vi "getClaseEstadistica.vi"(0 "claseEstadistica in":refnum<class "claseEstadistica.lvclass">, 3 "error in":errorcluster) -> (7 "claseEstadistica out":refnum<class "claseEstadistica.lvclass">, 8 "dataReading":T1, 10 "error out":errorcluster)   [LabVIEW 2014, in "claseEstadistica.lvclass"]
uses:
  claseEstadistica.lvclass
  claseEstadistica.lvclass/claseEstadistica.ctl
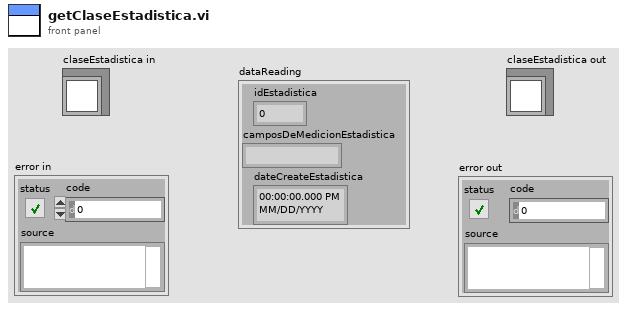
[diagram p1: front panel]
types:
  T1 = cluster{"idEstadistica":dbl, "camposDeMedicionEstadistica":string, "dateCreateEstadistica":timestamp}
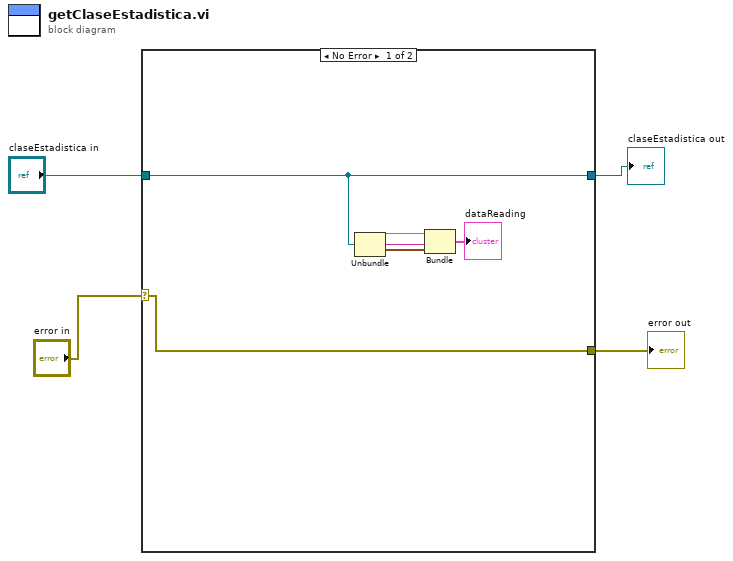
[diagram p0: block diagram]
diagram:
  n1 = case shown="No Error" "error in" {
    selector: "error in" -> [w10 w12]
    tunnel: [w10 w12] -> w3
    tunnel: "claseEstadistica in" -> [w9 w11]
    tunnel: [w9 w11] -> w1
    frame No Error {
      n2 = Unbundle(w9) -> (w8:dbl, w7:string, w6:timestamp)
      n3 = Bundle("idEstadistica"=w8, "camposDeMedicionEstadistica"=w7, "dateCreateEstadistica"=w6) -> (→"dataReading":T1)  [unwired: 1 in]
    }
    frame Error {
    }
  }
  "claseEstadistica out" <- w1
  "error out" <- w3
